vi "Filter Disconnect Waveforms.vi"(8 "error in (no error)":errorcluster, 11 "Waveform array in":waveform(dbl)[](array[waveform])=[{"t0"=timestamp(3637668094.8089256 s since 1904-01-01), "dt"=1.0, "Y"=[nan, nan, -244.9890895229809, -244.9890895229809, -244.9890895229809, -244.9890895229809, -244.9890895229809, -244.9890895229809, -244.9890895229809, -244.9890895229809, -244.9890895229809, -244.9890895229809, -244.9890895229809, -244.9890895229809, -244.9890895229809, -244.9890895229809, -244.9890895229809, -244.9890895229809, -244.9890895229809, -244.9890895229809, -244.9890895229809, -244.9890895229809, -244.9890895229809, -244.9890895229809, -244.9890895229809, -244.9890895229809, -244.9890895229809, -244.9890895229809, -244.9890895229809, -244.9890895229809, -244.9890895229809, -244.9890895229809, -244.9890895229809, -244.9890895229809, -244.9890895229809, -244.9890895229809, -244.9890895229809, -244.9890895229809, -244.9890895229809, -244.9890895229809], "attributes"=variant("NI_ChannelName"=variant(string "Temperature"))}, {"t0"=timestamp(3637668094.8089256 s since 1904-01-01), "dt"=1.0, "Y"=[nan, nan, 54.48011124083839, 54.48011124083839, 54.48011124083839, 54.48011124083839, 54.48011124083839, 54.82156418302147, 54.82156418302147, 54.82156418302147, 54.82156418302147, 54.82156418302147, 56.69630364911914, 56.69630364911914, 56.69630364911914, 56.69630364911914, 56.69630364911914, 57.46145038000977, 57.46145038000977, 57.46145038000977, 57.46145038000977, 57.46145038000977, 58.77816147939061, 58.77816147939061, 58.77816147939061, 58.77816147939061, 58.77816147939061, 60.19846638359926, 60.19846638359926, 60.19846638359926, 60.19846638359926, 60.19846638359926, 61.33543615829151, 61.33543615829151, 61.33543615829151, 61.33543615829151, 61.33543615829151, 62.82369632859256, 62.82369632859256, 62.82369632859256], "attributes"=variant("NI_ChannelName"=variant(string "Temperature_0"))}, {"t0"=timestamp(3637668094.8089256 s since 1904-01-01), "dt"=1.0, "Y"=[nan, nan, nan, nan, nan, nan, nan, nan, nan, nan, nan, nan, nan, nan, nan, nan, nan, nan, nan, nan, nan, nan, nan, nan, nan, nan, nan, nan, nan, nan, nan, nan, nan, nan, nan, nan, nan, nan, nan, nan], "attributes"=variant("NI_ChannelName"=variant(string "FD 1:Pump Flow"))}, {"t0"=timestamp(3637668094.8089256 s since 1904-01-01), "dt"=1.0, "Y"=[nan, nan, nan, nan, nan, nan, nan, nan, nan, nan, nan, nan, nan, nan, nan, nan, nan, nan, nan, nan, nan, nan, nan, nan, nan, nan, nan, nan, nan, nan, nan, nan, nan, nan, nan, nan, nan, nan, nan, nan], "attributes"=variant("NI_ChannelName"=variant(string "FD 1:PID2Out"))}, {"t0"=timestamp(3637668094.8089256 s since 1904-01-01), "dt"=1.0, "Y"=[nan, nan, nan, nan, nan, nan, nan, nan, nan, nan, nan, nan, nan, nan, nan, nan, nan, nan, nan, nan, nan, nan, nan, nan, nan, nan, nan, nan, nan, nan, nan, nan, nan, nan, nan, nan, nan, nan, nan, nan], "attributes"=variant("NI_ChannelName"=variant(string "FD 1:Input Device Disconnected"))}, {"t0"=timestamp(3637668094.8089256 s since 1904-01-01), "dt"=1.0, "Y"=[nan, nan, nan, nan, nan, nan, nan, nan, nan, nan, nan, nan, nan, nan, nan, nan, nan, nan, nan, nan, nan, nan, nan, nan, nan, nan, nan, nan, nan, nan, nan, nan, nan, nan, nan, nan, nan, nan, nan, nan], "attributes"=variant("NI_ChannelName"=variant(string "FD 1:Output Device Disconnected"))}, {"t0"=timestamp(3637668094.8089256 s since 1904-01-01), "dt"=1.0, "Y"=[nan, nan, nan, nan, nan, nan, nan, nan, nan, nan, nan, nan, nan, nan, nan, nan, nan, nan, nan, nan, nan, nan, nan, nan, nan, nan, nan, nan, nan, nan, nan, nan, nan, nan, nan, nan, nan, nan, nan, nan], "attributes"=variant("NI_ChannelName"=variant(string "FD 2:Pump Flow"))}, {"t0"=timestamp(3637668094.8089256 s since 1904-01-01), "dt"=1.0, "Y"=[nan, nan, nan, nan, nan, nan, nan, nan, nan, nan, nan, nan, nan, nan, nan, nan, nan, nan, nan, nan, nan, nan, nan, nan, nan, nan, nan, nan, nan, nan, nan, nan, nan, nan, nan, nan, nan, nan, nan, nan], "attributes"=variant("NI_ChannelName"=variant(string "FD 2:PID2Out"))}, {"t0"=timestamp(3637668094.8089256 s since 1904-01-01), "dt"=1.0, "Y"=[nan, nan, nan, nan, nan, nan, nan, nan, nan, nan, nan, nan, nan, nan, nan, nan, nan, nan, nan, nan, nan, nan, nan, nan, nan, nan, nan, nan, nan, nan, nan, nan, nan, nan, nan, nan, nan, nan, nan, nan], "attributes"=variant("NI_ChannelName"=variant(string "FD 2:Input Device Disconnected"))}, {"t0"=timestamp(3637668094.8089256 s since 1904-01-01), "dt"=1.0, "Y"=[nan, nan, nan, nan, nan, nan, nan, nan, nan, nan, nan, nan, nan, nan, nan, nan, nan, nan, nan, nan, nan, nan, nan, nan, nan, nan, nan, nan, nan, nan, nan, nan, nan, nan, nan, nan, nan, nan, nan, nan], "attributes"=variant("NI_ChannelName"=variant(string "FD 2:Output Device Disconnected"))}, {"t0"=timestamp(3637668094.8089256 s since 1904-01-01), "dt"=1.0, "Y"=[nan, nan, nan, nan, nan, nan, nan, nan, nan, nan, nan, nan, nan, nan, nan, nan, nan, nan, nan, nan, nan, nan, nan, nan, nan, nan, nan, nan, nan, nan, nan, nan, nan, nan, nan, nan, nan, nan, nan, nan], "attributes"=variant("NI_ChannelName"=variant(string "FD 3:Pump Flow"))}, {"t0"=timestamp(3637668094.8089256 s since 1904-01-01), "dt"=1.0, "Y"=[nan, nan, nan, nan, nan, nan, nan, nan, nan, nan, nan, nan, nan, nan, nan, nan, nan, nan, nan, nan, nan, nan, nan, nan, nan, nan, nan, nan, nan, nan, nan, nan, nan, nan, nan, nan, nan, nan, nan, nan], "attributes"=variant("NI_ChannelName"=variant(string "FD 3:Input Device Disconnected"))}, {"t0"=timestamp(3637668094.8089256 s since 1904-01-01), "dt"=1.0, "Y"=[nan, nan, nan, nan, nan, nan, nan, nan, nan, nan, nan, nan, nan, nan, nan, nan, nan, nan, nan, nan, nan, nan, nan, nan, nan, nan, nan, nan, nan, nan, nan, nan, nan, nan, nan, nan, nan, nan, nan, nan], "attributes"=variant("NI_ChannelName"=variant(string "FD 3:PID2Out"))}, {"t0"=timestamp(3637668094.8089256 s since 1904-01-01), "dt"=1.0, "Y"=[nan, nan, nan, nan, nan, nan, nan, nan, nan, nan, nan, nan, nan, nan, nan, nan, nan, nan, nan, nan, nan, nan, nan, nan, nan, nan, nan, nan, nan, nan, nan, nan, nan, nan, nan, nan, nan, nan, nan, nan], "attributes"=variant("NI_ChannelName"=variant(string "FD 3:Output Device Disconnected"))}]) -> (0 "error out":errorcluster, 3 "Waveform array out":waveform(dbl)[](array[waveform])=[{"t0"=timestamp(3637668094.8089256 s since 1904-01-01), "dt"=1.0, "Y"=[nan, nan, -244.9890895229809, -244.9890895229809, -244.9890895229809, -244.9890895229809, -244.9890895229809, -244.9890895229809, -244.9890895229809, -244.9890895229809, -244.9890895229809, -244.9890895229809, -244.9890895229809, -244.9890895229809, -244.9890895229809, -244.9890895229809, -244.9890895229809, -244.9890895229809, -244.9890895229809, -244.9890895229809, -244.9890895229809, -244.9890895229809, -244.9890895229809, -244.9890895229809, -244.9890895229809, -244.9890895229809, -244.9890895229809, -244.9890895229809, -244.9890895229809, -244.9890895229809, -244.9890895229809, -244.9890895229809, -244.9890895229809, -244.9890895229809, -244.9890895229809, -244.9890895229809, -244.9890895229809, -244.9890895229809, -244.9890895229809, -244.9890895229809], "attributes"=variant("NI_ChannelName"=variant(string "Temperature"))}, {"t0"=timestamp(3637668094.8089256 s since 1904-01-01), "dt"=1.0, "Y"=[nan, nan, 54.48011124083839, 54.48011124083839, 54.48011124083839, 54.48011124083839, 54.48011124083839, 54.82156418302147, 54.82156418302147, 54.82156418302147, 54.82156418302147, 54.82156418302147, 56.69630364911914, 56.69630364911914, 56.69630364911914, 56.69630364911914, 56.69630364911914, 57.46145038000977, 57.46145038000977, 57.46145038000977, 57.46145038000977, 57.46145038000977, 58.77816147939061, 58.77816147939061, 58.77816147939061, 58.77816147939061, 58.77816147939061, 60.19846638359926, 60.19846638359926, 60.19846638359926, 60.19846638359926, 60.19846638359926, 61.33543615829151, 61.33543615829151, 61.33543615829151, 61.33543615829151, 61.33543615829151, 62.82369632859256, 62.82369632859256, 62.82369632859256], "attributes"=variant("NI_ChannelName"=variant(string "Temperature_0"))}, {"t0"=timestamp(3637668094.8089256 s since 1904-01-01), "dt"=1.0, "Y"=[nan, nan, nan, nan, nan, nan, nan, nan, nan, nan, nan, nan, nan, nan, nan, nan, nan, nan, nan, nan, nan, nan, nan, nan, nan, nan, nan, nan, nan, nan, nan, nan, nan, nan, nan, nan, nan, nan, nan, nan], "attributes"=variant("NI_ChannelName"=variant(string "FD 1:Pump Flow"))}, {"t0"=timestamp(3637668094.8089256 s since 1904-01-01), "dt"=1.0, "Y"=[nan, nan, nan, nan, nan, nan, nan, nan, nan, nan, nan, nan, nan, nan, nan, nan, nan, nan, nan, nan, nan, nan, nan, nan, nan, nan, nan, nan, nan, nan, nan, nan, nan, nan, nan, nan, nan, nan, nan, nan], "attributes"=variant("NI_ChannelName"=variant(string "FD 1:PID2Out"))}, {"t0"=timestamp(3637668094.8089256 s since 1904-01-01), "dt"=1.0, "Y"=[nan, nan, nan, nan, nan, nan, nan, nan, nan, nan, nan, nan, nan, nan, nan, nan, nan, nan, nan, nan, nan, nan, nan, nan, nan, nan, nan, nan, nan, nan, nan, nan, nan, nan, nan, nan, nan, nan, nan, nan], "attributes"=variant("NI_ChannelName"=variant(string "FD 2:Pump Flow"))}, {"t0"=timestamp(3637668094.8089256 s since 1904-01-01), "dt"=1.0, "Y"=[nan, nan, nan, nan, nan, nan, nan, nan, nan, nan, nan, nan, nan, nan, nan, nan, nan, nan, nan, nan, nan, nan, nan, nan, nan, nan, nan, nan, nan, nan, nan, nan, nan, nan, nan, nan, nan, nan, nan, nan], "attributes"=variant("NI_ChannelName"=variant(string "FD 2:PID2Out"))}, {"t0"=timestamp(3637668094.8089256 s since 1904-01-01), "dt"=1.0, "Y"=[nan, nan, nan, nan, nan, nan, nan, nan, nan, nan, nan, nan, nan, nan, nan, nan, nan, nan, nan, nan, nan, nan, nan, nan, nan, nan, nan, nan, nan, nan, nan, nan, nan, nan, nan, nan, nan, nan, nan, nan], "attributes"=variant("NI_ChannelName"=variant(string "FD 3:Pump Flow"))}, {"t0"=timestamp(3637668094.8089256 s since 1904-01-01), "dt"=1.0, "Y"=[nan, nan, nan, nan, nan, nan, nan, nan, nan, nan, nan, nan, nan, nan, nan, nan, nan, nan, nan, nan, nan, nan, nan, nan, nan, nan, nan, nan, nan, nan, nan, nan, nan, nan, nan, nan, nan, nan, nan, nan], "attributes"=variant("NI_ChannelName"=variant(string "FD 3:PID2Out"))}])   [LabVIEW 2018, in "TDMS Log.lvlib"]
uses:
  TDMS Log.lvlib
panel:
  out "Channel Names":string[](array[string])=["Temperature", "Temperature_0", "FD 1:Pump Flow", "FD 1:PID2Out", "FD 2:Pump Flow", "FD 2:PID2Out", "FD 3:Pump Flow", "FD 3:PID2Out"]
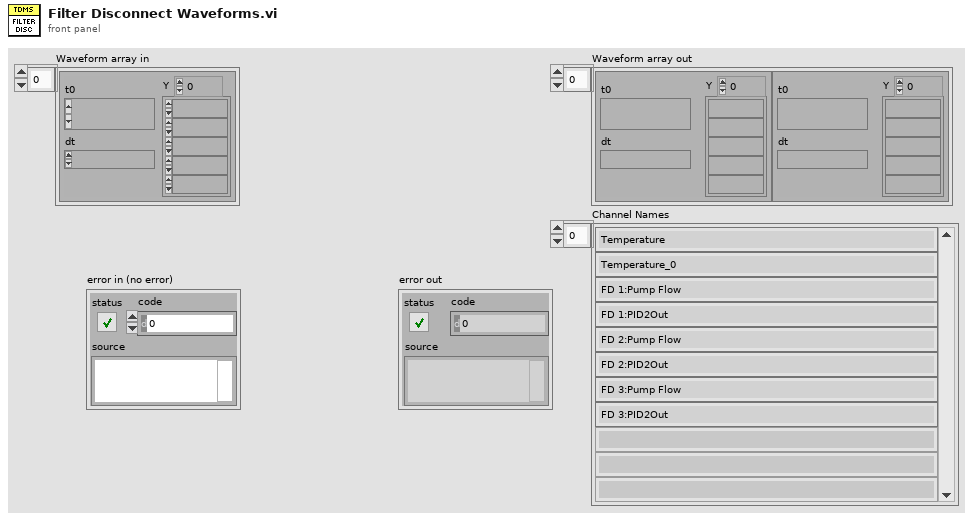
[diagram p1: front panel]
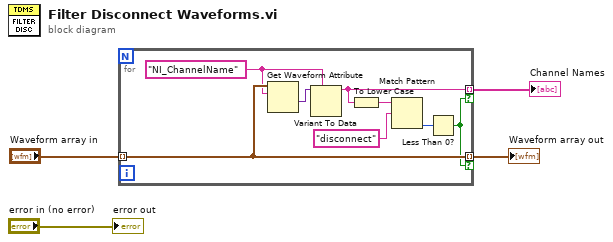
[diagram p0: block diagram]
diagram:
  n1 = for {
    tunnel: "Waveform array in" -> [w12] mode=indexing
    tunnel: [w12] -> w3 mode=indexing if=w5
    tunnel: [w6] -> w2 mode=indexing if=w5
    w10 = "NI_ChannelName" ("name")
    n2 = Get Waveform Attribute(6:w10, 7:w12) -> (1:w11:variant)  [unwired: 2 in, 3 out]
    n3 = Variant To Data(type=w10, Variant=w11) -> (data=w6:string)  [unwired: 1 in, 1 out]
    n4 = To Lower Case(string=w6) -> (all lower case string=w9:string)
    n5 = Match Pattern(string=w9, regular expression="disconnect" ("name")) -> (offset past match=w7:i32)  [unwired: 1 in, 3 out]
    n6 = Less Than 0?(x=w7) -> (x < 0?=w5:bool)
  }
  "Waveform array out" <- w3
  "Channel Names" <- w2
  "error out" <- "error in (no error)"
